vi "Get Table Alais Columns Name.vi"(8 "error in (no error)":errorcluster, 10 "TableName":string, 11 "HostDB in":refnum<class "SQLite.lvclass">) -> (0 "error out":errorcluster, 1 "Alais_ColunmsList":string[](array[string]), 2 "Table_ColunmsList":string[](array[string]), 3 "HostDB out":refnum<class "SQLite.lvclass">, 4 "TableName List":string[](array[string]))   [LabVIEW 2017, in "SQLite.lvclass"]
doc: "only for the results.db table. which have the alais columns name."
uses:
  SQLite.lvclass
  \\vmware-host\Shared Folders/D/Dev/NJAL/OP140/OP140_NJAL_valve_EOL_Test_20210806/Source_Public/DataBase/Top DB/TopDBClass.lvclass
  <userlib>/LabSQL/LabSQL.lvlib
  <userlib>/sushu/sushu.lvlib
panel:
  out "String":string
  out "DB Data Type":T1(array[ring])
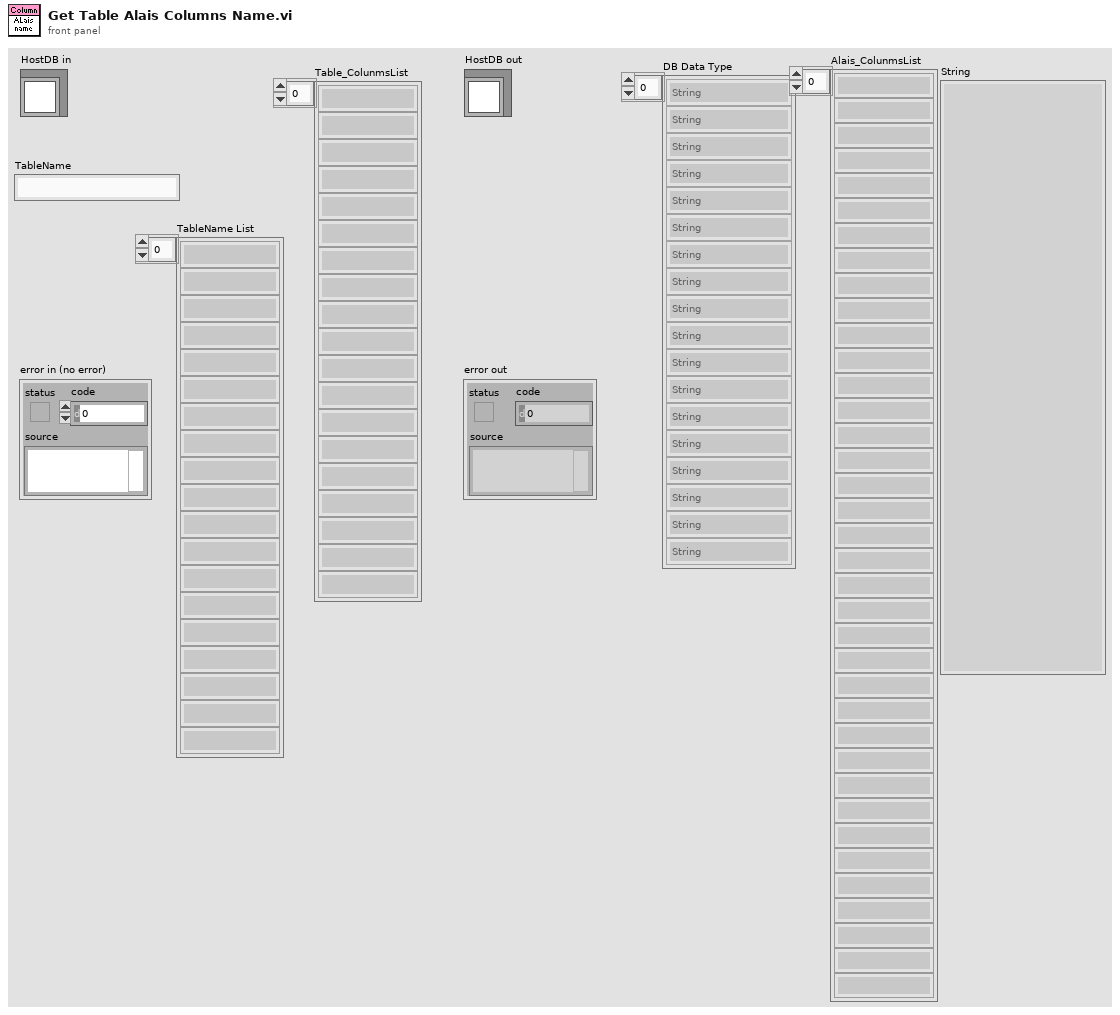
[diagram p1: front panel]
types:
  T1 = enum16{"String", "Long (I32)", "Single (SGL)", "Double (DBL)", "Date/Time", "Binary"}[]
  T2 = enum16{"Other", "SQL2008", "SQLite", "Access", "MySQL"}
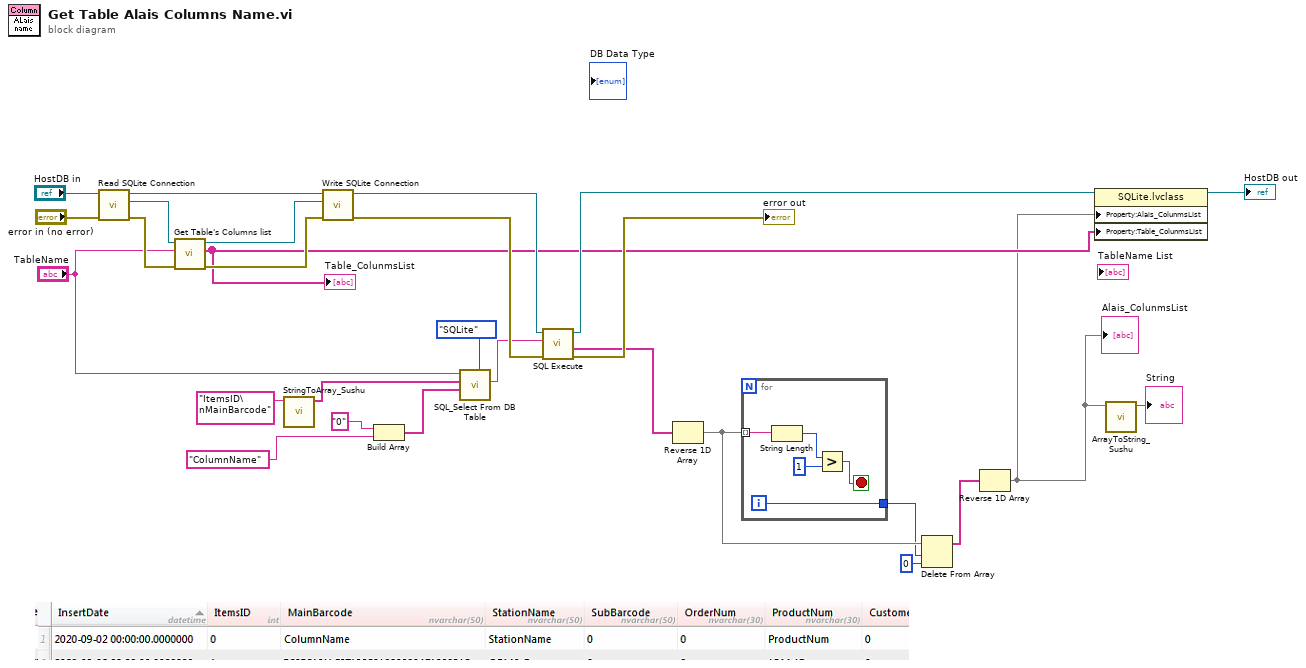
[diagram p0: block diagram]
diagram:
  n1 = call-dynamic "Read SQLite Connection.vi"("error in (no error)"="error in (no error)", "SQLite in"="HostDB in") -> ("error out"=w26:errorcluster, "SQLite.lvlib:Connection"=w27:refnum<class "Connection.lvclass">, "SQLite out"=w24:refnum<class "SQLite.lvclass">)  [unwired: 7 in]
  n2 = call <userlib>:"Get Table's Columns list.vi"("error in (no error)"=w26, "TabelName"="TableName", "SQLite Connection in"=w27) -> ("error out"=w25:errorcluster, "Column Names"=w15:string[], "SQLite Connection out"=w21:refnum<class "Connection.lvclass">)  [unwired: 5 in, 1 out]
  "Table_ColunmsList" <- w15
  n3 = call <userlib>:"StringToArray_Sushu.vi"("State Queue"="ItemsID\nMainBarcode") -> ("Array"=w8:string[])  [unwired: 8 in, 2 out]
  n4 = call-dynamic "Write SQLite Connection.vi"("error in (no error)"=w25, "SQLite.lvlib:Connection"=w21, "SQLite in"=w24) -> ("error out"=w18:errorcluster, "SQLite out"=w20:refnum<class "SQLite.lvclass">)  [unwired: 7 in]
  n5 = Build Array("0" ("element"), "ColumnName" ("State Queue")) -> (w9:string[])
  n6 = call <userlib>:"SQL_Select From DB Table.vi"("DB Type"=T2."SQLite", "ColumnsValue"=w9, "ColumnsNameList"=w8, "TableName"="TableName") -> ("Select SQL CMD"=w11:string)  [unwired: 7 in]
  n7 = call-dynamic "SQL Execute.vi"("error in (no error)"=w18, "Command Text"=w11, "HostDB in"=w20) -> ("error out"=→"error out":errorcluster, "FirstRow"=w5:string[], "HostDB out"=w19:refnum<class "SQLite.lvclass">)  [unwired: 4 in, 2 out]
  n8 = Reverse 1D Array(array=w5) -> (reversed array=w4:string[])
  n9 = for {
    tunnel: w4 -> [w33] mode=indexing
    tunnel: [w29] -> w3
    i -> [w29]
    stop <- w30 stop-if-true
    n10 = String Length(string=w33) -> (length=w32:i32)
    n11 = Greater?(x=w32, y=1) -> (0:w30:bool)
  }
  n12 = Delete From Array(array=w4, length=w3, index=0) -> (array with subset deleted=w1:string[])  [unwired: 1 out]
  n13 = Reverse 1D Array(array=w1) -> (reversed array=w14:string[])
  "Alais_ColunmsList" <- w14
  n14 = property class="SQLite.lvclass"(reference=w19, "Property:Alais_ColunmsList"=w14, "Property:Table_ColunmsList"=w15) -> (reference out=→"HostDB out":refnum<class "SQLite.lvclass">)  [unwired: 1 in, 1 out]
  n15 = call <userlib>:"ArrayToString_Sushu.vi"("Array"=w14) -> ("String"=→"String":string)  [unwired: 10 in]
